vi "Z Aux Trans Stringto Int.vi"(8 "error in (no error)":errorcluster caption="错误输入（无错误）", 9 "pivlaue":i32, 10 "inumes":i32, 11 "pstringin":string) -> (0 "error out":errorcluster caption="错误输出", 1 "pivlaue out":i32, 3 "function return":i32)   [LabVIEW 2015, in "zauxdll.lvlib"]
doc: "int32 __stdcall ZAux_TransStringtoInt(const char* pstringin, int inumes, int* pivlaue);"
uses:
  zauxdll.lvlib
  zauxdll.dll
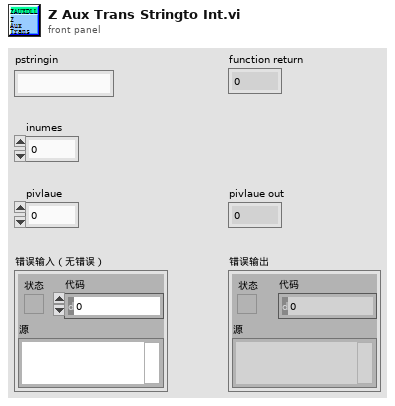
[diagram p1: front panel]
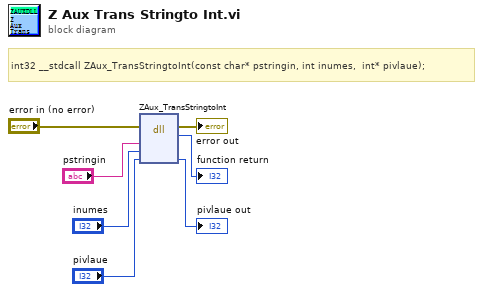
[diagram p0: block diagram]
diagram:
  # "int32 __stdcall ZAux_TransStringtoInt(const char* pstringin, int inumes,  int* pivlaue);"
  n1 = dll-call lib="C:/Users/VIC/Desktop/GOGORO_Oringnal - Panasonic/system/LLB/zmotion/zaux/zauxdll.*" fn="ZAux_TransStringtoInt"(error in="error in (no error)", "pstringin"="pstringin", "inumes"="inumes", "pivlaue"="pivlaue") -> (error out=→"error out":errorcluster, →"function return":i32, "pivlaue"=→"pivlaue out":i32)  [unwired: 4 in, 1 out]
